vi "config crosslink test.vi"() -> (0 "error out":errorcluster, 1 "Pass":bool, 2 "Editor crosslinked?":bool, 3 "Runtime crosslinked?":bool)   [LabVIEW 2015, in "Sequencer Module tests.lvlib"]
uses:
  Sequencer Module tests.lvlib
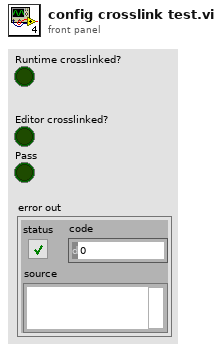
[diagram p1: front panel]
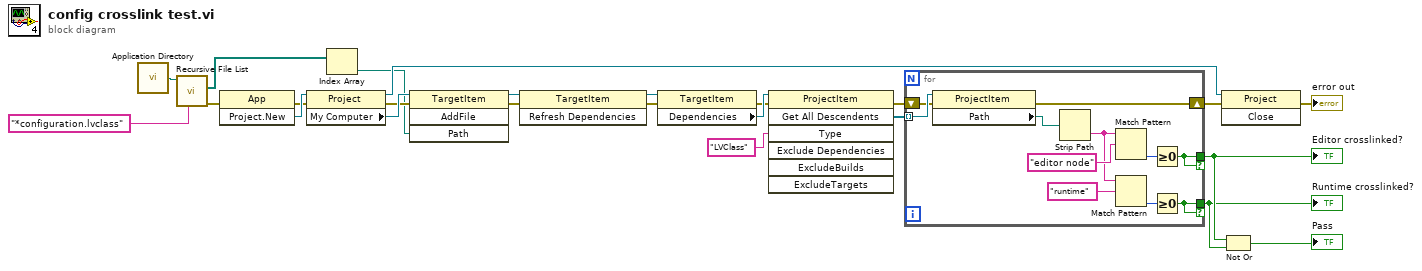
[diagram p0: block diagram]
diagram:
  n1 = call <vilib>:"Application Directory.vi"() -> ("Application Directory"=w8:path)
  n2 = call <vilib>:"Recursive File List.vi"("pattern"="*configuration.lvclass", "Folder Path"=w8) -> ("error out"=w4:errorcluster, "All Files in Dir"=w6:path[])  [unwired: 5 in, 3 out]
  n3 = invoke class="App" method="Project.New"(error in=w4) -> (error out=w18:errorcluster, "Project:New"=w21:refnum<vi>)  [unwired: 2 in, 1 out]
  n4 = property class="Project"(reference=w21, error in=w18) -> (reference out=w12:refnum<vi>, error out=w19:errorcluster, "My Computer"=w20:refnum<vi>)
  n5 = Index Array(array=w6) -> (element=w5:path)  [unwired: 1 in]
  n6 = invoke class="TargetItem" method="AddFile"(reference=w20, error in=w19, "Path"=w5) -> (reference out=w17:refnum<vi>, error out=w15:errorcluster)  [unwired: 1 in, 2 out]
  n7 = invoke class="TargetItem" method="Refresh Dependencies"(reference=w17, error in=w15) -> (reference out=w16:refnum<vi>, error out=w14:errorcluster)  [unwired: 1 in, 1 out]
  n8 = property class="TargetItem"(reference=w16, error in=w14) -> (error out=w10:errorcluster, "Dependencies"=w23:refnum<vi>)  [unwired: 1 out]
  n9 = invoke class="ProjectItem" method="Get All Descendents"(reference=w23, error in=w10, "Type"="LVClass") -> (error out=w11:errorcluster, "All Descendents"=w22:refnum<vi>[])  [unwired: 4 in, 5 out]
  n10 = for {
    tunnel: w22 -> [w35] mode=indexing
    shift-right: [w34] -> w13
    shift-left: w11 -> [w33]
    tunnel: [w26] -> w3 if=w26
    tunnel: [w25] -> w2 if=w25
    n11 = property class="ProjectItem"(reference=w35, error in=w33) -> (error out=w34:errorcluster, "Path"=w32:path)  [unwired: 1 out]
    n12 = Strip Path(path=w32) -> (name=w29:string)  [unwired: 1 out]
    n13 = Match Pattern(string=w29, regular expression="editor node") -> (offset past match=w30:i32)  [unwired: 1 in, 3 out]
    n14 = Match Pattern(string=w29, regular expression="runtime") -> (offset past match=w27:i32)  [unwired: 1 in, 3 out]
    n15 = Greater Or Equal To 0?(x=w30) -> (x >= 0?=w26:bool)
    n16 = Greater Or Equal To 0?(x=w27) -> (x >= 0?=w25:bool)
  }
  "Editor crosslinked?" <- w3
  "Runtime crosslinked?" <- w2
  n17 = invoke class="Project" method="Close"(reference=w12, error in=w13) -> (error out=→"error out":errorcluster)  [unwired: 1 in, 2 out]
  n18 = Not Or(1:w2, 2:w3) -> (0:→"Pass":bool)
